vi "GenINI_Wire_Top_And_Bottom.vi"(8 "error in":errorcluster, 10 "vi 2 ref":refnum<vi>, 11 "vi 1 ref":refnum<vi>) -> (0 "error out":errorcluster, 2 "vi 2 ref dup":refnum<vi>, 3 "vi 1 ref dup":refnum<vi>)   [LabVIEW 2009]
doc: "Wire top and bottom of the 4815 unrotated connector on two VI's."
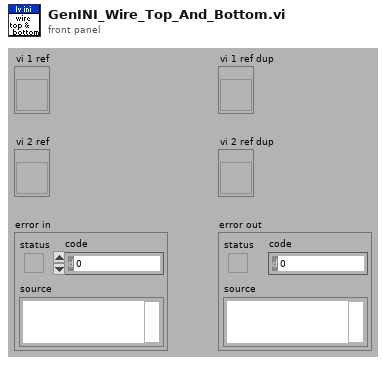
[diagram p1: front panel]
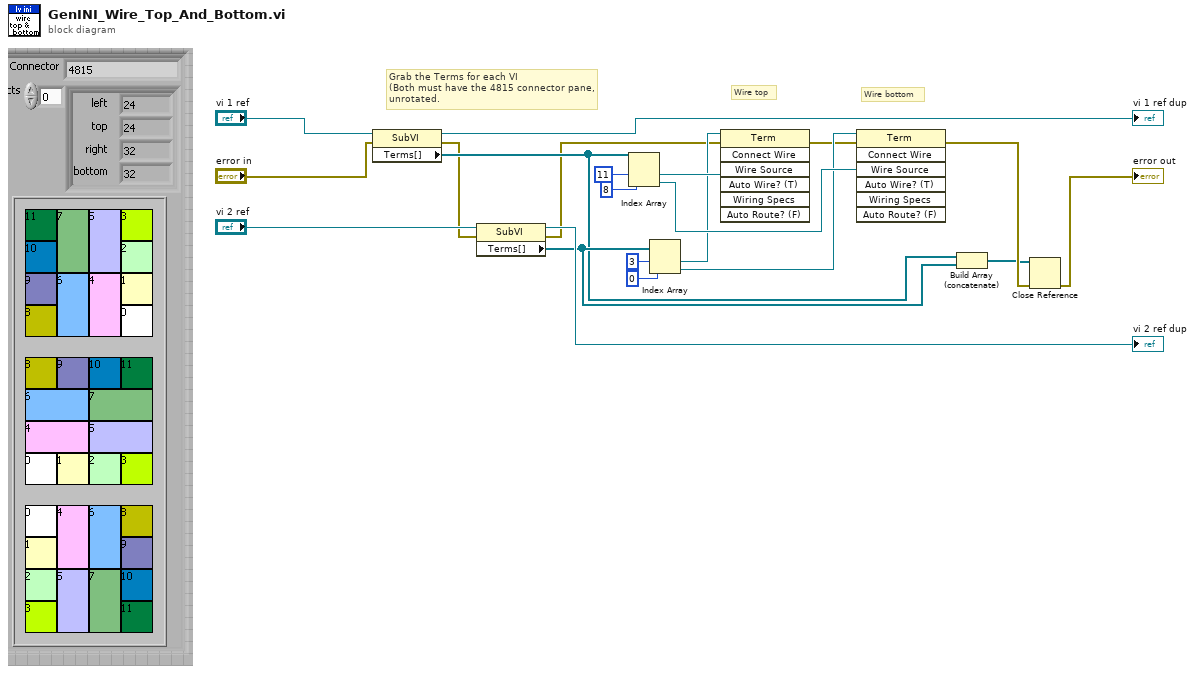
[diagram p0: block diagram]
diagram:
  # "Wire bottom"
  # "Wire top"
  # "Grab the Terms for each VI\n(Both must have the 4815 connector pane,\nunrotated."
  n1 = property class="SubVI"(reference="vi 1 ref", error in="error in") -> (reference out=→"vi 1 ref dup":refnum<vi>, error out=w2:errorcluster, "Terms[]"=w16:refnum<vi>[])
  n2 = property class="SubVI"(reference="vi 2 ref", error in=w2) -> (reference out=→"vi 2 ref dup":refnum<vi>, error out=w1:errorcluster, "Terms[]"=w17:refnum<vi>[])
  n3 = Index Array(array=w16, index #1=11 ("index"), index #2=8 ("index")) -> (element #1=w11:refnum<vi>, element #2=w20:refnum<vi>)
  n4 = Index Array(array=w17, index #1=3 ("index"), index #2=0 ("index")) -> (element #1=w10:refnum<vi>, element #2=w15:refnum<vi>)
  n5 = invoke class="Term" method="Connect Wire"(reference=w10, error in=w1, "Wire Source"=w11) -> (error out=w12:errorcluster)  [unwired: 4 in, 6 out]
  n6 = invoke class="Term" method="Connect Wire"(reference=w15, error in=w12, "Wire Source"=w20) -> (error out=w19:errorcluster)  [unwired: 4 in, 6 out]
  n7 = Build Array (concatenate)(w16, w17) -> (w18:refnum<vi>[])
  n8 = Close Reference(reference=w18, error in (no error)=w19) -> (error out=→"error out":errorcluster)
